vi "test step by step.vi"() -> ()   [LabVIEW 2016]
uses:
  <vilib>/userdefined/High Color/nirio_resource_hc.ctl
  <vilib>/FPGAPlugInAG/cRIO-9033/niLvFpga_Open_cRIO-9033.vi
  <vilib>/rvi/interface/common/dynamic/niFpgaDynamicAddResources.vi
  <vilib>/CANopenLib/CANOPEN.llb/CANopen Emergency Create.vi
  <vilib>/CANopenLib/CANOPEN.llb/CANopen Emergency Read.vi
  <vilib>/CANopenLib/CANOPEN.llb/CANopen Emergency Close.vi
  <vilib>/CANopenLib/CANOPEN.llb/CANopen SDO Create.vi
  <vilib>/CANopenLib/CANOPEN.llb/CANopen SDO Write [U8].vi
  <vilib>/CANopenLib/CANOPEN.llb/CANopen SDO Close.vi
  <vilib>/rvi/interface/nirviOpenFPGA/nirviOpenFPGA.xnode
  Users/s163601/Desktop/05-28/FPGA Bitfiles/project_FPGATarget_MainFPGA_S9ZLErdeBuw.lvbitx
  Users/s163601/Desktop/05-28/RT/FPGA/MainFPGA.vi
panel:
  in  "Node ID":u8 min=1 max=127 step=1
  out "emergency message":T1 {"manufacturer specific error field" format="%.0x"; "error register" format="%.0x"; "error code" format="%.0x"}
  in  "error in (no error)":errorcluster
  in  "counter overflow value":u8=5
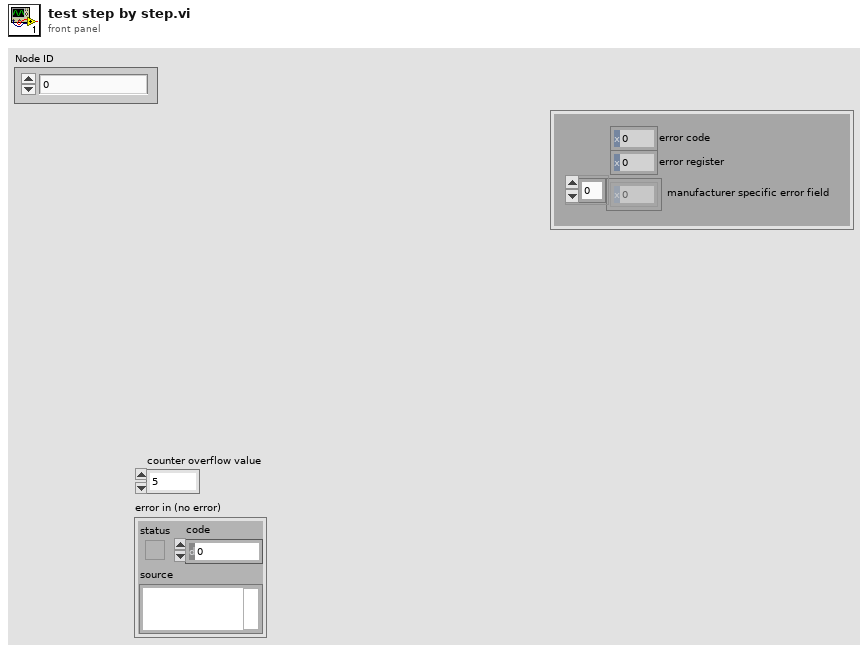
[diagram p1: front panel]
types:
  T1 = cluster{"error code":u16, "error register":u8, "manufacturer specific error field":u8[]}
  T2 = typedef "nirio_resource_hc.ctl" = tag
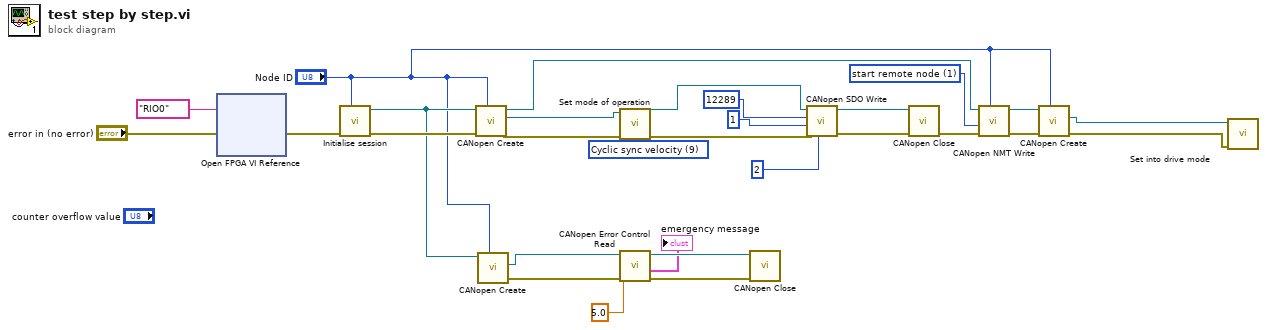
[diagram p0: block diagram]
diagram:
  w8 = i8 9 items=["Induction VF – testing purposes only"=-5, "Aligning rotor position"=-4, "Current stepper – testing purposes only "=-3, "Voltage stepper – testing purposes only"=-2, "Voltage constant angle – testing purposes only"=-1, "No mode"=0, "Cyclic sync position"=8, "Cyclic sync velocity"=9, "Cyclic sync torque"=10] ("Mode of operation")
  w22 = u16 1 items=["start remote node"=1, "stop remote node"=2, "enter pre-operational"=128, "reset node"=129, "reset communication"=130] ("command")
  n1 = xnode ("Open FPGA VI Reference")("error in"="error in (no error)", "resource name"=T2 "RIO0") -> ("error out"=w28:errorcluster)  [unwired: 1 out]
  n2 = call "Initialise session.vi"("Node ID"="Node ID", "error in"=w28) -> ("error out"=w26:errorcluster, "interface object out"=w10:refnum<k20>)  [unwired: 7 in, 1 out]
  n3 = call-poly <vilib>:"CANopen Create.vi"("node-ID"="Node ID", "error in (no error)"=w26, "interface object in"=w10) -> ("error out"=w4:errorcluster, "SDO object out"=w5:refnum<k20>, "interface object out"=w18:refnum<k20>)  [unwired: 6 in]
  n4 = call-poly <vilib>:"CANopen Create.vi"("node-ID"="Node ID", "interface object in"=w10) -> ("error out"=w14:errorcluster, "emergency object out"=w15:refnum<k20>)  [unwired: 7 in, 1 out]
  n5 = call "Set mode of operation.vi"("Mode of operation"=w8, "error in (no error)"=w4, "SDO object in"=w5) -> ("error out"=w7:errorcluster, "SDO object out"=w6:refnum<k20>)  [unwired: 6 in, 1 out]
  n6 = call-poly <vilib>:"CANopen Error Control Read.vi"("error in (no error)"=w14, "timeout (0s)"=5.0, "emergency object in"=w15) -> ("error out"=w13:errorcluster, "emergency message"=→"emergency message":T1, "emergency object out"=w12:refnum<k20>)  [unwired: 4 in, 2 out]
  n7 = call-poly <vilib>:"CANopen Close.vi"("error in (no error)"=w13, "emergency object in"=w12) -> ()  [unwired: 9 in, 1 out]
  n8 = call-poly <vilib>:"CANopen SDO Write.vi"("U8 data"=2 ("I32 data"), "error in (no error)"=w7, "object sub-index (0)"=1 ("I32 data"), "object index"=u16 12289, "SDO object in"=w6) -> ("error out"=w21:errorcluster, "SDO object out"=w20:refnum<k20>)  [unwired: 4 in, 1 out]
  n9 = call-poly <vilib>:"CANopen Close.vi"("error in (no error)"=w21, "SDO object in"=w20) -> ("error out"=w19:errorcluster)  [unwired: 9 in]
  n10 = call <vilib>:"CANopen NMT Write.vi"("node-ID (0)"="Node ID", "error in (no error)"=w19, "command"=w22, "interface object in"=w18) -> ("error out"=w16:errorcluster, "interface object out"=w17:refnum<k20>)  [unwired: 6 in]
  n11 = call-poly <vilib>:"CANopen Create.vi"("node-ID"="Node ID", "error in (no error)"=w16, "interface object in"=w17) -> ("error out"=w2:errorcluster, "SDO object out"=w3:refnum<k20>)  [unwired: 6 in, 1 out]
  n12 = call "Set into drive mode.vi"("error in (no error)"=w2, "SDO object in"=w3) -> ()  [unwired: 8 in, 2 out]
